vi "add_image_lossless.vi"(6 "values":string[](array[string]), 7 "keys":string[](array[string]), 8 "error in (no error)":errorcluster, 9 "timestamp_ns":i64, 10 "img":u16[][](array[numeric]), 11 "h264_file_handle":u64) -> (0 "error out":errorcluster, 3 "h264_file_handle":u64)   [LabVIEW 2011, in "librir.lvlib"]
uses:
  librir.lvlib
  libs/video_io.dll
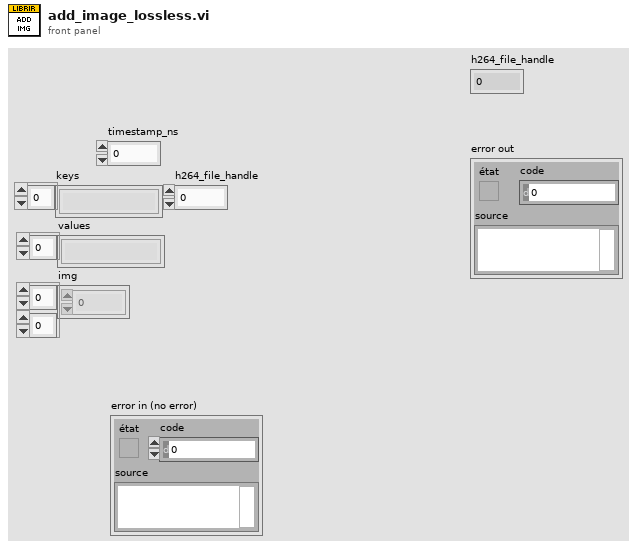
[diagram p1: front panel]
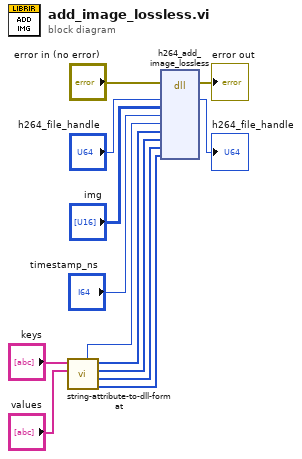
[diagram p0: block diagram]
diagram:
  n1 = call "string-attribute-to-dll-format.vi"("values"="values", "keys"="keys") -> ("values_length"=w3:i32[], "values"=w4:i8[], "keys_length"=w5:i32[], "keys"=w6:i8[], "attribute count"=w2:i32)  [unwired: 5 in]
  n2 = dll-call lib="G:/librir/src/labview/libs/video_io.dll" fn="h264_add_image_lossless"(error in="error in (no error)", "h264_file_handle"="h264_file_handle", "img"="img", "timestamp_ns"="timestamp_ns", "attribute_count"=w2, "keys"=w6, "keys_length"=w5, "values"=w4, "values_length"=w3) -> (error out=→"error out":errorcluster, "h264_file_handle"=→"h264_file_handle":u64)  [unwired: 10 in, 1 out]
